vi "Dequeue AppEvent Element.vi"(8 "Error In":errorcluster, 9 "Timeout":i32, 11 "EventLog in":refnum<class "EventLog.lvclass">) -> (0 "Error Out":errorcluster, 1 "Timed out?":bool, 3 "EventLog out":refnum<class "EventLog.lvclass">)   [LabVIEW 2019, in "EventLog.lvlib" / "EventLog.lvclass"]
uses:
  EventLog.lvclass
  EventLog.lvclass/EventLog.ctl
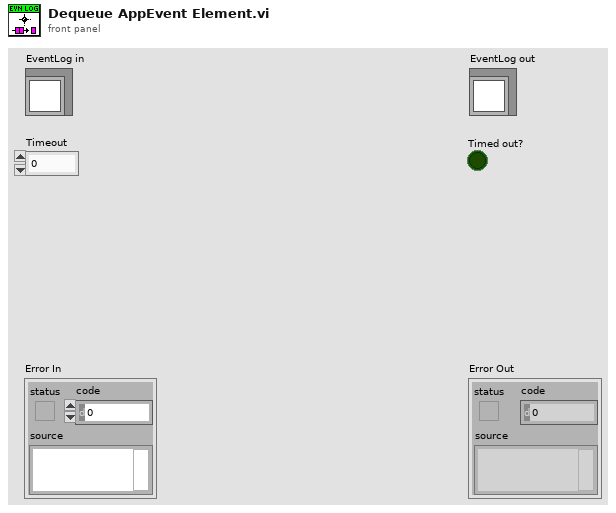
[diagram p1: front panel]
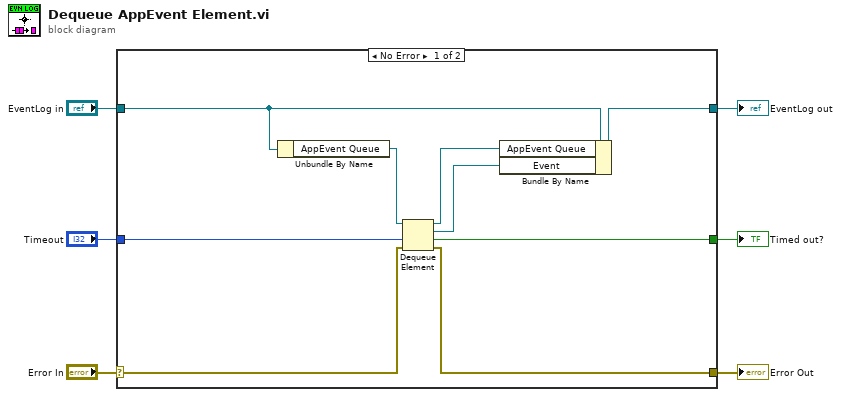
[diagram p0: block diagram]
diagram:
  n1 = case shown="No Error" "Error In" {
    selector: "Error In" -> [w13 w17]
    tunnel: [w12 w17] -> w5
    tunnel: [w11 w16] -> w3
    tunnel: "EventLog in" -> [w15 w16]
    tunnel: [w8 _] -> w2
    tunnel: "Timeout" -> [w7 _]
    frame No Error {
      n2 = Unbundle By Name(w15) -> ("AppEvent Queue"=w14:refnum<queue>)
      n3 = Dequeue Element(queue=w14, timeout in ms (-1)=w7, error in (no error)=w13) -> (queue out=w9:refnum<queue>, element=w10:refnum<class "Events.lvclass">, timed out?=w8:bool, error out=w12:errorcluster)
      n4 = Bundle By Name(cluster=w15, "AppEvent Queue"=w9, "Event"=w10) -> (w11:refnum<class "EventLog.lvclass">)
    }
    frame Error {
    }
  }
  "Error Out" <- w5
  "EventLog out" <- w3
  "Timed out?" <- w2
